vi "Day5Part2.vi"(10 "UpdatedPages":string="75,47,61,53,29\n97,61,53,29,13\n75,29,13\n75,97,47,61,53\n61,13,29\n97,13,75,29,47", 11 "OrderingRules":string="47|53\n97|13\n97|61\n97|47\n75|29\n61|13\n75|53\n29|13\n97|29\n53|29\n61|53\n97|53\n61|29\n47|13\n75|47\n97|75\n47|61\n75|61\n47|29\n75|13\n53|13") -> (3 "Result":i64)   [LabVIEW 2024]
uses:
  <vilib>/Utility/miscctls.llb/LVMapReplaceAction.ctl
panel:
  out "MidNumbers":i64[](array[numeric])
  out "Map":map{i32, i32[]}(c390)
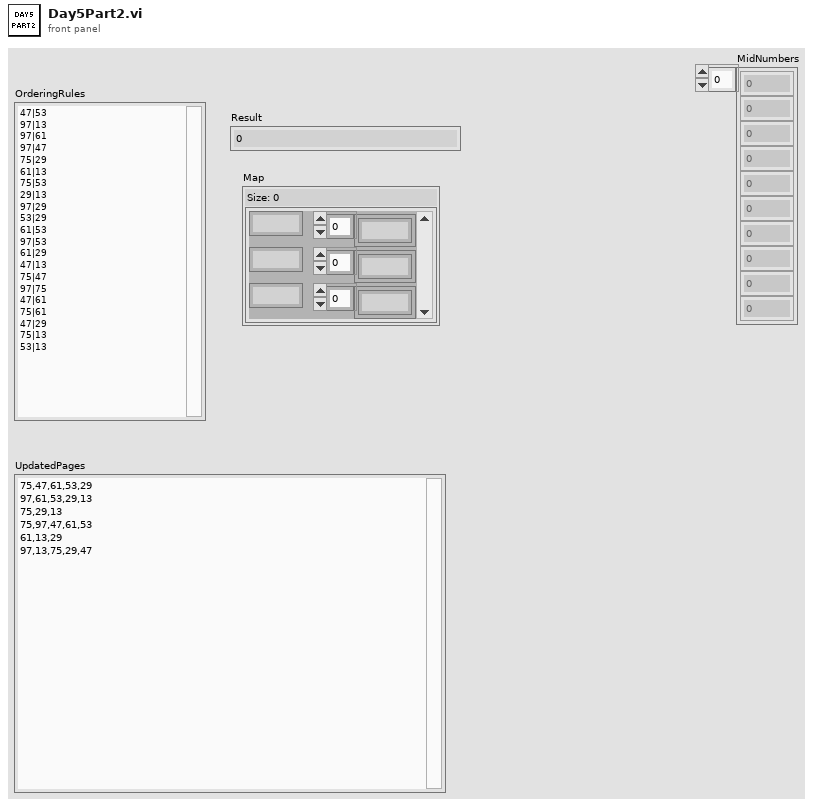
[diagram p1: front panel]
types:
  T1 = typedef "LVMapReplaceAction.ctl" = enum32{"Modify Entry only if found", "Add or Modify Entry", "Delete Entry"}
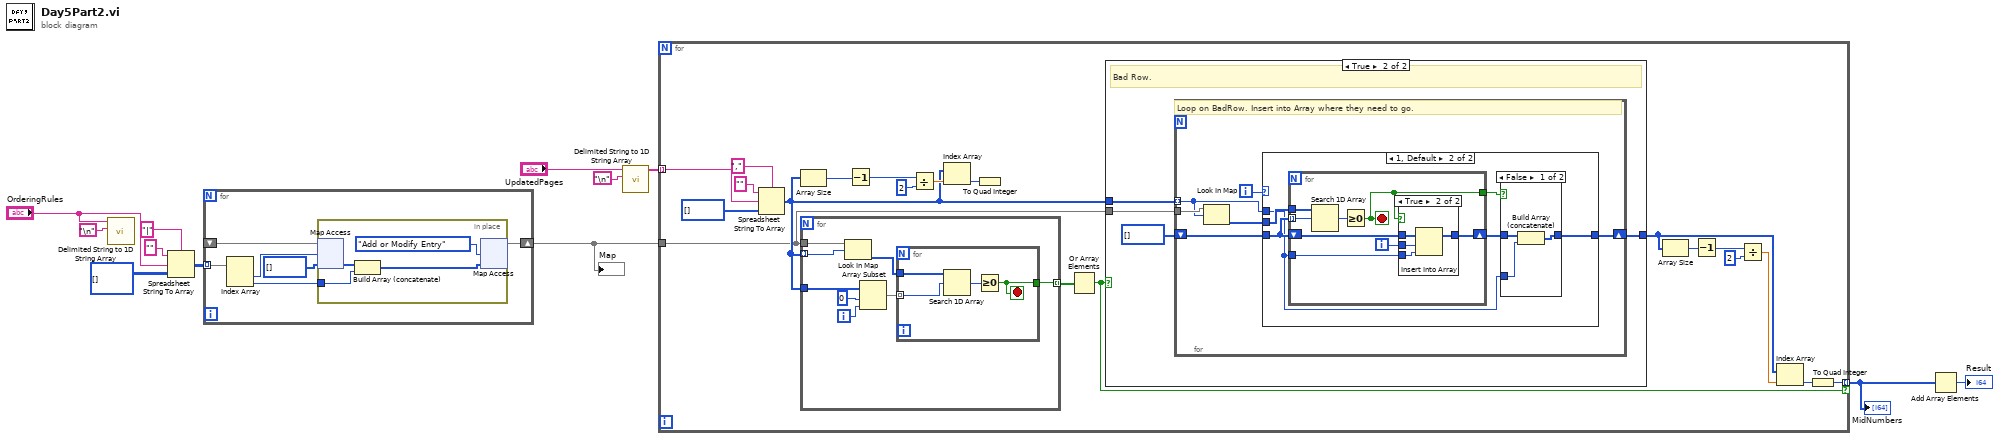
[diagram p0: block diagram]
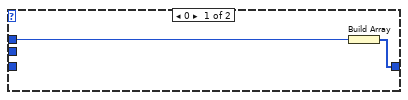
[diagram p3: hidden frame]
diagram:
  n1 = call <vilib>:"Delimited String to 1D String Array.vi"("delimiter"="\n", "delimited string"="OrderingRules") -> ()  [unwired: 9 in, 1 out]
  n2 = Spreadsheet String To Array(delimiter (Tab)="|", format string="", spreadsheet string="OrderingRules", array type (2D Dbl)=i32[][] []) -> (array=w4:i32[][])
  n3 = for {
    tunnel: w4 -> [w18] mode=indexing
    shift-right: [w13] -> w3
    shift-left: _ -> [w16]
    n4 = Index Array(array=w18) -> (element #1=w17:i32, element #2=w14:i32)  [unwired: 2 in]
    n5 = in-place {
      in-place-border: w14 -> [w21]
      n6 = in-place-map #1(w16, w17, i32[] []) -> (w22:i32[])  [unwired: 1 out]
      n7 = Build Array (concatenate)(w22, w21) -> (w20:i32[])
      n8 = in-place-map #1(w20, LVMapReplaceAction."Add or Modify Entry" ("action")) -> (w13:map{i32, i32[]})  [unwired: 2 out]
    }
  }
  "Map" <- w3
  n9 = call <vilib>:"Delimited String to 1D String Array.vi"("delimiter"="\n", "delimited string"="UpdatedPages") -> ("string array"=w9:string[])  [unwired: 9 in]
  n10 = for {
    tunnel: w9 -> [w42] mode=indexing
    tunnel: w3 -> [w31]
    tunnel: [w25] -> w2 mode=indexing if=w24
    n11 = Spreadsheet String To Array(delimiter (Tab)=",", format string="", spreadsheet string=w42, array type (2D Dbl)=i32[] []) -> (array=w32:i32[])
    n12 = Array Size(array=w32) -> (size(s)=w37:i32)
    n13 = for {
      tunnel: w32 -> [w85] mode=indexing
      tunnel: w31 -> [w78]
      tunnel: w32 -> [w79]
      tunnel: [w80] -> w38 mode=indexing
      i -> [w84]
      n14 = Look In Map(map=w78, key=w85) -> (value=w81:i32[])  [unwired: 1 in, 1 out]
      n15 = Array Subset(array=w79, index=0, length=w84) -> (w82:i32[])
      n16 = for {
        tunnel: w82 -> [w88] mode=indexing
        tunnel: w81 -> [w89]
        tunnel: [w86] -> w80
        stop <- w86 stop-if-true
        n17 = Search 1D Array(1D array=w89, element=w88) -> (index of element=w87:i32)  [unwired: 1 in]
        n18 = Greater Or Equal To 0?(x=w87) -> (x >= 0?=w86:bool)
      }
    }
    n19 = Decrement(x=w37) -> (x-1=w36:i32)
    n20 = Divide(x=w36, y=2) -> (x/y=w34:dbl)
    n21 = Index Array(array=w32, index=w34) -> (element=w33:i32)
    n22 = To Quad Integer(1:w33) -> ()  [unwired: 1 out]
    n23 = Or Array Elements(Boolean array=w38) -> (logical OR=w24:bool)
    n24 = case shown="True" w24 {
      tunnel: w32 -> [_ w46]
      tunnel: w31 -> [_ w44]
      tunnel: [_ w43] -> w23
      frame False {
      }
      frame True {
        # "Bad Row."
        n25 = for {
          tunnel: w46 -> [w49] mode=indexing
          shift-right: [w48] -> w43
          shift-left: i32[] [] -> [w52]
          tunnel: w44 -> [w51]
          i -> [w47]
          # "Loop on BadRow. Insert into Array where they need to go."
          n26 = Look In Map(map=w51, key=w49) -> (value=w50:i32[])  [unwired: 1 in, 1 out]
          n27 = case shown="1, Default" w47 {
            tunnel: w52 -> [_ w59]
            tunnel: w50 -> [_ w60]
            tunnel: w49 -> [w54 w55]
            tunnel: [w53 w56] -> w48
            frame 0 {
              n28 = Build Array(w54) -> (w53:i32[])
            }
            frame 1, Default {
              n29 = for {
                tunnel: w59 -> [w71] mode=indexing
                tunnel: w60 -> [w72]
                shift-right: [w66] -> w57
                shift-left: w59 -> [w68]
                tunnel: w55 -> [w67]
                tunnel: [w65] -> w58
                i -> [w69]
                stop <- w65 stop-if-true
                n30 = Search 1D Array(1D array=w72, element=w71) -> (index of element=w70:i32)  [unwired: 1 in]
                n31 = Greater Or Equal To 0?(x=w70) -> (x >= 0?=w65:bool)
                n32 = case shown="True" w65 {
                  tunnel: w69 -> [_ w74]
                  tunnel: w68 -> [w73 w77]
                  tunnel: w67 -> [_ w76]
                  tunnel: [w73 w75] -> w66
                  frame False {
                  }
                  frame True {
                    n33 = Insert Into Array(array=w77, index=w74, new element=w76) -> (w75:i32[])
                  }
                }
              }
              n34 = case shown="False" w58 {
                tunnel: w57 -> [w63 w64]
                tunnel: [w62 w64] -> w56
                tunnel: w55 -> [w61 _]
                frame False {
                  n35 = Build Array (concatenate)(w63, w61) -> (w62:i32[])
                }
                frame True {
                }
              }
            }
          }
        }
      }
    }
    n36 = Array Size(array=w23) -> (size(s)=w30:i32)
    n37 = Decrement(x=w30) -> (x-1=w29:i32)
    n38 = Divide(x=w29, y=2) -> (x/y=w27:dbl)
    n39 = Index Array(array=w23, index=w27) -> (element=w26:i32)
    n40 = To Quad Integer(1:w26) -> (0:w25:i64)
  }
  "MidNumbers" <- w2
  n41 = Add Array Elements(numeric array=w2) -> (sum=→"Result":i64)
